vi "PictureControl_Draw Text at Point.vi"(0 "text orientation":T1(ring), 4 "BG color(transparent)":u32(colorbox)=16777216, 5 "[user-specified font]":T5={"Font Name:"="", "Size"=12, "Strikeout?"=FALSE, "Italic?"=FALSE, "Underline?"=FALSE, "Outline?"=FALSE, "Shadow?"=FALSE, "Bold?"=FALSE}, 6 "text color(black)":u32(colorbox), 7 "desired font(Application)":T4(ring)=enum."Application Font", 8 "text":string, 9 "alignment(left, top)":T3, 10 "origin":cluster{"x":i16, "y":i16}, 11 "picture":picture) -> (2 "text rect":T2, 3 "new picture":picture)   [LabVIEW 2020]
doc: "Draws a string into a picture."
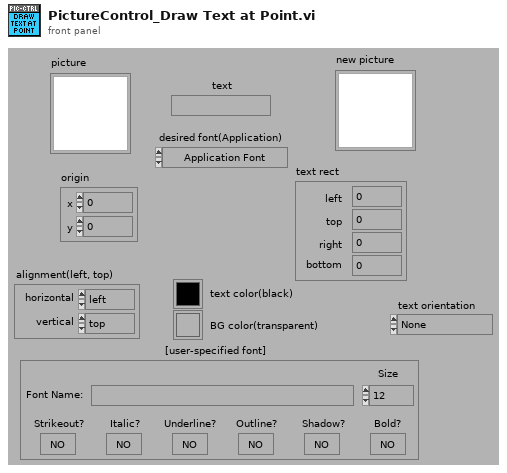
[diagram p1: front panel]
types:
  T1 = enum16{"None", "Stacked", "Clockwise", "Counterclockwise"}
  T2 = cluster{"left":i16, "top":i16, "right":i16, "bottom":i16}
  T3 = cluster{"horizontal":enum16{"left", "center", "right"}, "vertical":enum16{"top", "center", "bottom"}}
  T4 = enum16{"User-specified Font", "Application Font", "System Font", "Dialog Font"}
  T5 = cluster{"Font Name:":string, "Size":i16, "Strikeout?":bool, "Italic?":bool, "Underline?":bool, "Outline?":bool, "Shadow?":bool, "Bold?":bool}
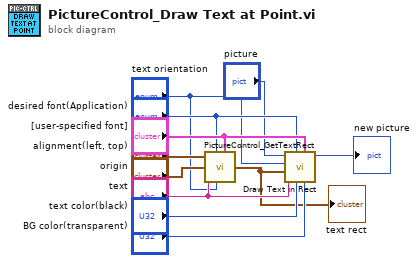
[diagram p0: block diagram]
diagram:
  n1 = call "PictureControl_GetTextRect.vi"("alignment(left, top)"="alignment(left, top)", "desired font(Application)"="desired font(Application)", "origin(0,0)"="origin", "text"="text", "text orientation"="text orientation", "[user-specified font]"="[user-specified font]") -> ("rect"=w4:T2)  [unwired: 3 in]
  "text rect" <- w4
  n2 = call <vilib>:"Draw Text in Rect.vi"("BG color(transparent)"="BG color(transparent)", "[user-specified font]"="[user-specified font]", "text color(black)"="text color(black)", "desired font(Application)"="desired font(Application)", "text"="text", "rect"=w4, "text orientation"="text orientation", "picture"="picture") -> ("new picture"=→"new picture":picture)  [unwired: 3 in]
